vi "Hypergeometric Moments.vi"(8 "n":i32=20, 9 "k":i32=30, 10 "M":i32=100) -> (0 "error":i32, 2 "variance":dbl=3.3939393939393936, 3 "mean":dbl=6.0)   [LabVIEW 2017, in "NI_Gmath.lvlib"]
doc: "Returns the expected mean and variance of the random variate X, where X describes the selected distribution type. You must manually select the polymorphic instance to use."
uses:
  NI_Gmath.lvlib
  st_error_code.ctl
panel:
  # "Hypergeometric Moments"
  # "size of population"
  # "items"
  # "samples drawn"
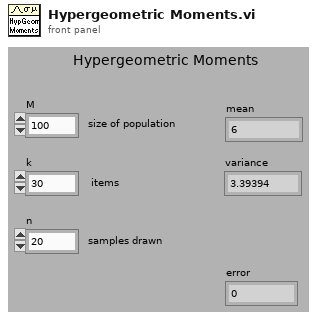
[diagram p1: front panel]
types:
  T1 = typedef "NI_Gmath.lvlib/st_error_code.ctl" = i32
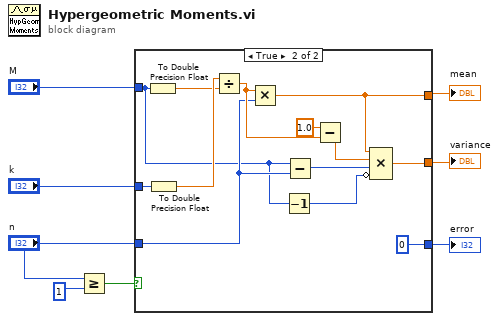
[diagram p0: block diagram]
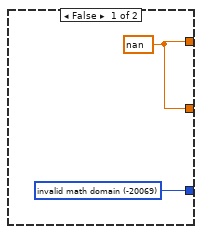
[diagram p2: hidden frame]
diagram:
  n1 = Greater Or Equal?(x="n", y=1 ("n = samples drawn")) -> (x >= y?=w6:bool)
  n2 = case shown="True" w6 {
    tunnel: [w10 w18] -> w5
    tunnel: [w10 w11] -> w8
    tunnel: [w9 0 ("error")] -> w4
    tunnel: "n" -> [_ w15]
    tunnel: "k" -> [_ w22]
    tunnel: "M" -> [_ w13]
    frame False {
      w9 = T1 -20069 items=["invalid math domain"=-20069, "Fourier interpolation size m >= n"=-20070, "empty array"=-20003] ("stat interp error code")
      w10 = nan
    }
    frame True {
      n3 = To Double Precision Float(number=w13) -> (double precision float=w16:dbl)
      n4 = To Double Precision Float(number=w22) -> (double precision float=w20:dbl)
      n5 = Divide(x=w20, y=w16) -> (x/y=w19:dbl)
      n6 = Multiply(x=w19, y=w15) -> (x*y=w18:dbl)
      n7 = Decrement(x=w13) -> (x-1=w12:i32)
      n8 = Subtract(x=w13, y=w15) -> (x-y=w14:i32)
      n9 = Subtract(x=1.0, y=w19) -> (x-y=w17:dbl)
      n10 = Compound Arithmetic op=MULTIPLY(w18, w17, w14, invert w12) -> (w11:dbl)
    }
  }
  "mean" <- w5
  "error" <- w4
  "variance" <- w8
